vi "ep_Convert Spectra to Pair Points.vi"(8 "error in (no error)":errorcluster, 11 "spectra":T1) -> (0 "error out":errorcluster, 1 "min frequency":dbl, 2 "max frequency":dbl, 3 "spectra points":T2)   [LabVIEW 2014, in "NI_EP_Motor Monitoring.lvlib"]
uses:
  <vilib>/addons/Electrical Power/Motor Monitoring/NI_EP_Motor Monitoring.lvlib
  <vilib>/Analysis/1siggen.llb/Ramp Pattern by Delta.vi
  <vilib>/Analysis/NI_AALBase.lvlib
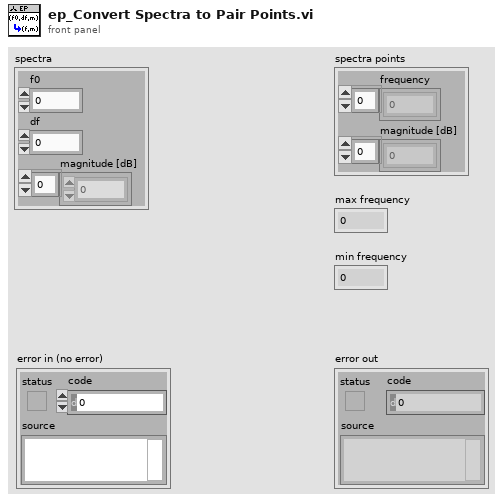
[diagram p1: front panel]
types:
  T1 = cluster{"f0":dbl, "df":dbl, "magnitude [dB]":dbl[]}
  T2 = cluster{"frequency":dbl[], "magnitude [dB]":dbl[]}
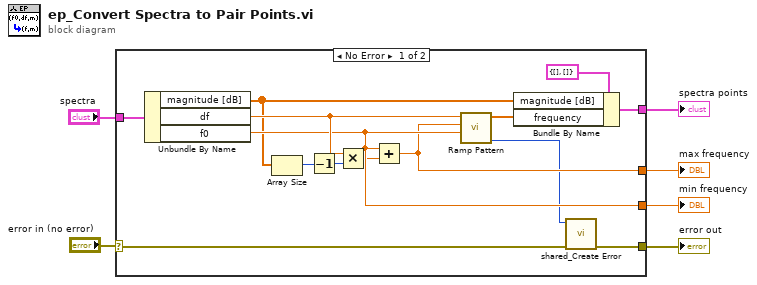
[diagram p0: block diagram]
diagram:
  n1 = case shown="No Error" "error in (no error)" {
    selector: "error in (no error)" -> [w8 w21]
    tunnel: [w17 _] -> w6
    tunnel: [w16 _] -> w5
    tunnel: [w12 _] -> w4
    tunnel: "spectra" -> [w10 _]
    tunnel: [w9 w21] -> w1
    frame No Error {
      n2 = Unbundle By Name(w10) -> ("magnitude [dB]"=w14:dbl[], "df"=w18:dbl, "f0"=w17:dbl)
      n3 = Array Size(array=w14) -> (size(s)=w20:i32)
      n4 = Decrement(x=w20) -> (x-1=w19:i32)
      n5 = Multiply(x=w18, y=w19) -> (x*y=w15:dbl)
      n6 = Add(x=w17, y=w15) -> (x+y=w16:dbl)
      n7 = call-poly <vilib>:"Ramp Pattern.vi"("start"=w17, "end"=w16, "delta"=w18) -> ("error"=w7:i32, "Ramp Pattern"=w13:dbl[])  [unwired: 6 in, 1 out]
      n8 = Bundle By Name(cluster=T2 {"frequency"=[], "magnitude [dB]"=[]} ("spectra points"), "magnitude [dB]"=w14, "frequency"=w13) -> (w12:T2)
      n9 = call <vilib>:"shared_Create Error.vi"("error in (no error)"=w8, "error code (0)"=w7) -> ("error out"=w9:errorcluster)  [unwired: 9 in]
    }
    frame Error {
    }
  }
  "min frequency" <- w6
  "max frequency" <- w5
  "spectra points" <- w4
  "error out" <- w1
